vi "axisFont.vi"(8 "Error In":errorcluster, 10 "axisId":T1 items=["YLeft", "YRight", "XBottom", "XTop"], 11 "QwtPlot In":refnum<class "QwtPlot.lvclass">) -> (0 "Error Out":errorcluster, 2 "Value":refnum<class "QFont.lvclass">, 3 "QwtPlot Out":refnum<class "QwtPlot.lvclass">)   [LabVIEW 2014, in "QwtPlot.lvclass"]
doc: "LabVIEW-specific documentation is not yet available. See <b>https://qwt.sourceforge.io/class_qwt_plot.html#axisFont</b>"
uses:
  QwtPlot.lvclass
  Qt GUI/QFont/QFont.lvclass
  QwtAxis/Position.ctl
  LQ Core/LQIdentity/LQIdentity.lvclass/LQIdentity.ctl
  LQ Core/LQSerialData/LQSerialData.lvclass/LQSerialData.ctl
  LQ Core/LQ Core.lvlib
  LQ Core/LQIdentity/LQIdentity.lvclass
  LQ Core/LQSerialData/LQSerialData.lvclass
  QwtAxis/QwtAxis.lvlib
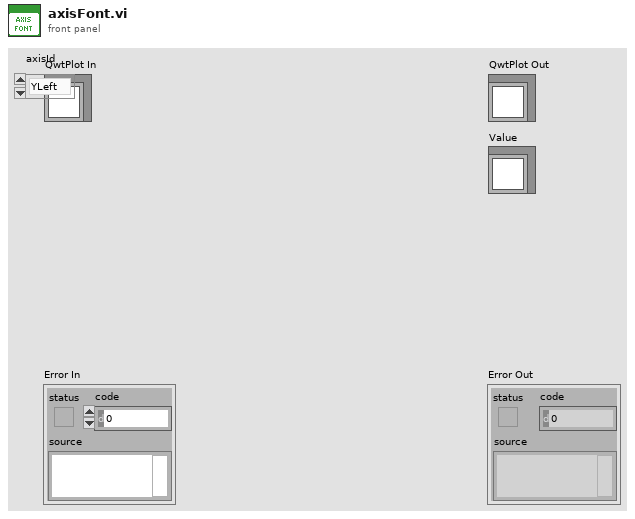
[diagram p1: front panel]
types:
  T1 = typedef "QwtAxis.lvlib/Position.ctl" = i32
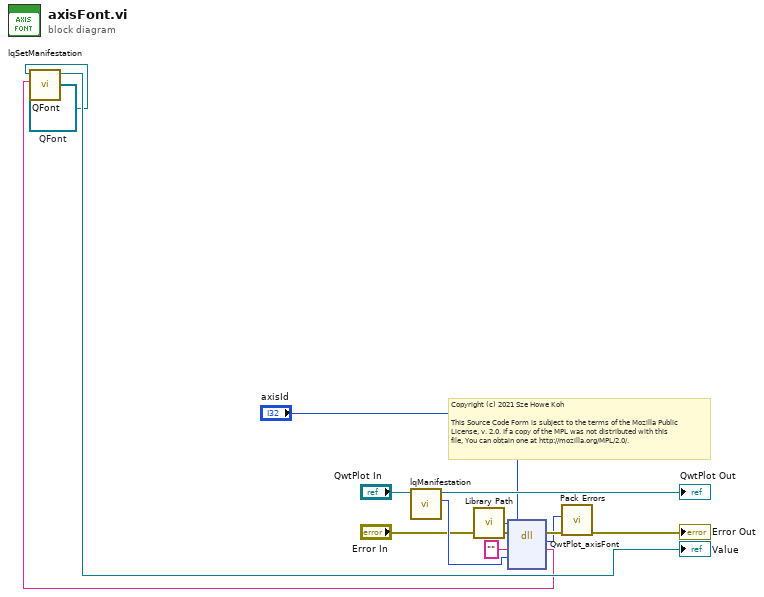
[diagram p0: block diagram]
diagram:
  w2 = refnum<class "QFont.lvclass"> refnum  # QFont
  # "Copyright (c) 2021 Sze Howe Koh\n\nThis Source Code Form is subject to the terms of the Mozilla Public\nLicense, v. 2.0. If a copy of the MPL was not distributed with this\nfile, You can obtain one at http://mozilla.org/MPL/2.0/."
  n1 = call "lqManifestation.vi"("LQIdentity in"="QwtPlot In") -> ("Manifestation"=w9:u64, "LQIdentity out"=→"QwtPlot Out":refnum<class "QwtPlot.lvclass">)  [unwired: 9 in]
  n2 = call "Library Path.vi"() -> ("Library Path"=w10:path)
  n3 = dll-call lib="?" fn="QwtPlot_axisFont"(path in=w10, error in="Error In", "_retVal"="" ("retVal"), "_instance"=w9, "axisId"="axisId") -> (error out=w7:errorcluster, w5:i32, "_retVal"=w3:string)  [unwired: 3 in, 1 out]
  n4 = call "lqSetManifestation.vi"("Manifestation"=w3, "LQSerialData in"=w2) -> ("LQSerialData out"=→"Value":refnum<class "QFont.lvclass">)  [unwired: 8 in, 1 out]
  n5 = call "Pack Errors.vi"("Error In"=w7, "Error Code"=w5) -> ("Error Out"=→"Error Out":errorcluster)  [unwired: 9 in]
